vi "Autonomous Independent.vi"() -> ()   [LabVIEW 2012]
doc: "This VI is called when autonomous begins, and will automatically be terminated when autonomous ends. You can carry out timed or sensor driven robot movement independently without needing to return to the caller."
uses:
  AutoInstruction.ctl
  AutoInstructArray.ctl
  Sally_Dashboard_2013/DBNameEnum.ctl
  Robot Global Data.vi
  AutoEnum.ctl
panel:
  in  "DefaultBackupAuto":dbl[](array[numeric])=[2390.0, 30.0, 3.0, 4.0, 1000.0, 0.0]
  in  "AutoBackup":T1
  in  "AutoDefault":T1=[{"Distance/Angle"=30.0, "Speed"=2390.0, "Action"=enum."Aim", "NumFrisbees"=0}, {"Distance/Angle"=5.0, "Speed"=0.0, "Action"=enum."Wait", "NumFrisbees"=0}, {"Distance/Angle"=0.0, "Speed"=0.0, "Action"=enum."Shoot", "NumFrisbees"=4}]
  out "ValueFromDashboard":T1
  in  "Desired steady state (no PID)":dbl=0.5
  in  "Use PID AutoDrive":bool=TRUE
  in  "AutoInstructArray":T1=[{"Distance/Angle"=0.0, "Speed"=0.0, "Action"=enum."DriveForward", "NumFrisbees"=0}, {"Distance/Angle"=0.0, "Speed"=0.0, "Action"=enum."DriveForward", "NumFrisbees"=0}, {"Distance/Angle"=0.0, "Speed"=0.0, "Action"=enum."DriveForward", "NumFrisbees"=0}]
  in  "Instructions":T3(array[cluster])
  in  "Instruction Sequence":T4(array[cluster])
  in  "AutoInstruction":T2
  # "GLENN'S STUFF"
  # "ENUMS FOR\nSTRING UNFLATTENING"
  # "RPM"
  # "Angle"
  # "Wait (s)"
  # "ShootNum"
  # "Time (ms)"
  # "Drive Back Stuff"
  # "Motor Value"
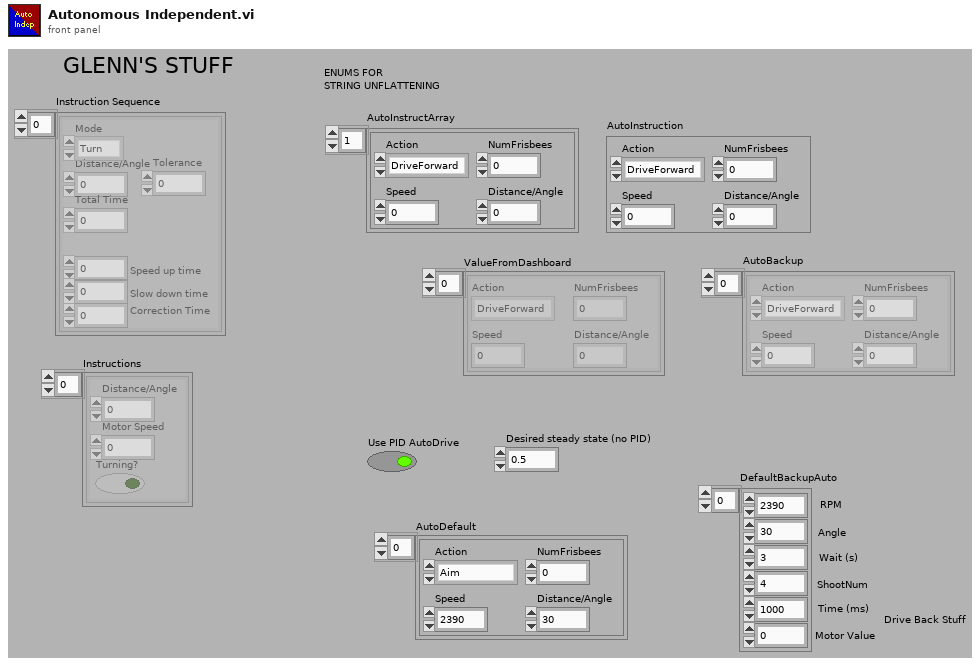
[diagram p1: front panel]
types:
  T1 = typedef "AutoInstructArray.ctl" = T2[]
  T2 = typedef "AutoInstruction.ctl" = cluster{"Distance/Angle":dbl, "Speed":dbl, "Action":enum16{"DriveForward", "Turn", "Aim", "Shoot", "Wait"}, "NumFrisbees":i32}
  T3 = cluster{"Distance/Angle":dbl, "Motor Speed":dbl, "Turning?":bool}[]
  T4 = cluster{"Distance/Angle":dbl, "Tolerance":dbl, "Total Time":dbl, "Mode":enum16{"Turn", "Drive"}, "Correction Time":dbl, "Speed up time":dbl, "Slow down time":dbl}[]
  T5 = typedef "DBNameEnum.ctl" = enum16{"AutoInstructions", "DriveLoopTime", "DriveAlignLSLeft", "DriveAlignLSRight", "Use2DriveAlign", "ClimbLS", "LauncherAngleMatches", "FrameworkVersion", "sLauncherAngle", "LauncherTargetAngle", "sLauncherRPM", "LauncherTargetRPM", "sDriveDistance", "LauncherMotorValue", "PullbackTol", "FireTol", "LauncherRPMTol", "LauncherAngleTol", "InitialWait", "WaitBetweenLaunch", "AnglePresets", "RPMPresets", "UseAngleEncoder", "UseLauncherEncoder", "UseLauncherPID", "QSWaitBeforeFire", "QSWaitBeforeRetract", "AngleForwardValue", "AngleBackwardValue", "UseClusterArray", "BackupAuto", "ReverseDriveIndicate", "HalfSpeedFactor"}
  T6 = typedef "WPI_EncoderDevRef.ctl" = cluster{"DevStatus":errorcluster, "EncoderIndex":T7, "CounterIndex":T8, "DistancePerCount":dbl, "Decoding Type":T9}
  T7 = typedef "FPGA_EncoderIdx.ctl" = enum8{"Enc 0", "Enc 1", "Enc 2", "Enc 3", "Invalid"}
  T8 = typedef "FPGA_CounterCtrSystemIndex.ctl" = enum8{"Ctr 0", "Ctr 1", "Ctr 2", "Ctr 3", "Ctr 4", "Ctr 5", "Ctr 6", "Ctr 7", "Invalid"}
  T9 = typedef "WPI_EncoderType.ctl" = enum16{"1x", "2x", "4x"}
  T10 = typedef "WPI_GyroDevRef.ctl" = cluster{"DevStatus":errorcluster, "Analog Module":T11, "Analog Channel":T12, "Offset":dbl, "Gain (VoltsPerDegree/Second)":dbl}
  T11 = typedef "FPGA_TypedefAnalogModule.ctl" = enum16{"Analog Module 1", "Analog Module 2"}
  T12 = typedef "FPGA_AIChannel.ctl" = enum8{"AI 1", "AI 2", "AI 3", "AI 4", "AI 5", "AI 6", "AI 7", "AI 8", "Invalid"}
  T13 = typedef "WPI_RobotDriveDevRef.ctl" = cluster{"DevStatus":errorcluster, "Motors[]":T14[], "Square Inputs":bool, "Max Output":dbl, "Isochronous":bool}
  T14 = typedef "WPI_MotorControlDeviceRef.ctl" = cluster{"DeviceStatus":errorcluster, "Type":enum16{"PWM", "CAN"}, "PWM":cluster{"Digital Module":T15, "PWM Channel":T16, "DeadBand":T17}, "CAN":cluster{"Device Number":u8, "Control Mode":T18, "Semaphore":T19, "Max Vout":dbl}, "Invert":bool, "TransformRef":T20, "InvTransformRef":T20}
  T15 = typedef "FPGA_TypedefDigitalModule.ctl" = enum16{"Digital Module 1", "Digital Module 2"}
  T16 = typedef "FPGA_DIOPWMChannel.ctl" = enum8{"PWM 1", "PWM 2", "PWM 3", "PWM 4", "PWM 5", "PWM 6", "PWM 7", "PWM 8", "PWM 9", "PWM 10", "Invalid"}
  T17 = typedef "WPI_PWMDeadband.ctl" = cluster{"Name":string, "maxPositivePwm":i32, "minPositivePwm":i32, "centerPwm":i32, "maxNegativePwm":i32, "minNegativePwm":i32, "angularRange":u16}
  T18 = typedef "WPI_CANJaguar_ControlMode.ctl" = enum8{"Percent VBus", "Current", "Speed", "Position", "Voltage"}
  T19 = typedef "Semaphore RefNum" = refnum<k1>
  T20 = typedef "WPI_PWMTransform_ConPane.ctl" = refnum<vi>
  T21 = typedef "AutoEnum.ctl" = enum16{"Disabled", "BackRight", "BackLeft", "CloseRight", "CloseLeft", "BehindPyramid"}
  T22 = enum16{"DriveForward", "Turn", "Aim", "Shoot", "Wait", "LauncherDown"}
  T23 = enum16{"DriveForward", "Turn", "Aim", "Shoot", "Wait"}
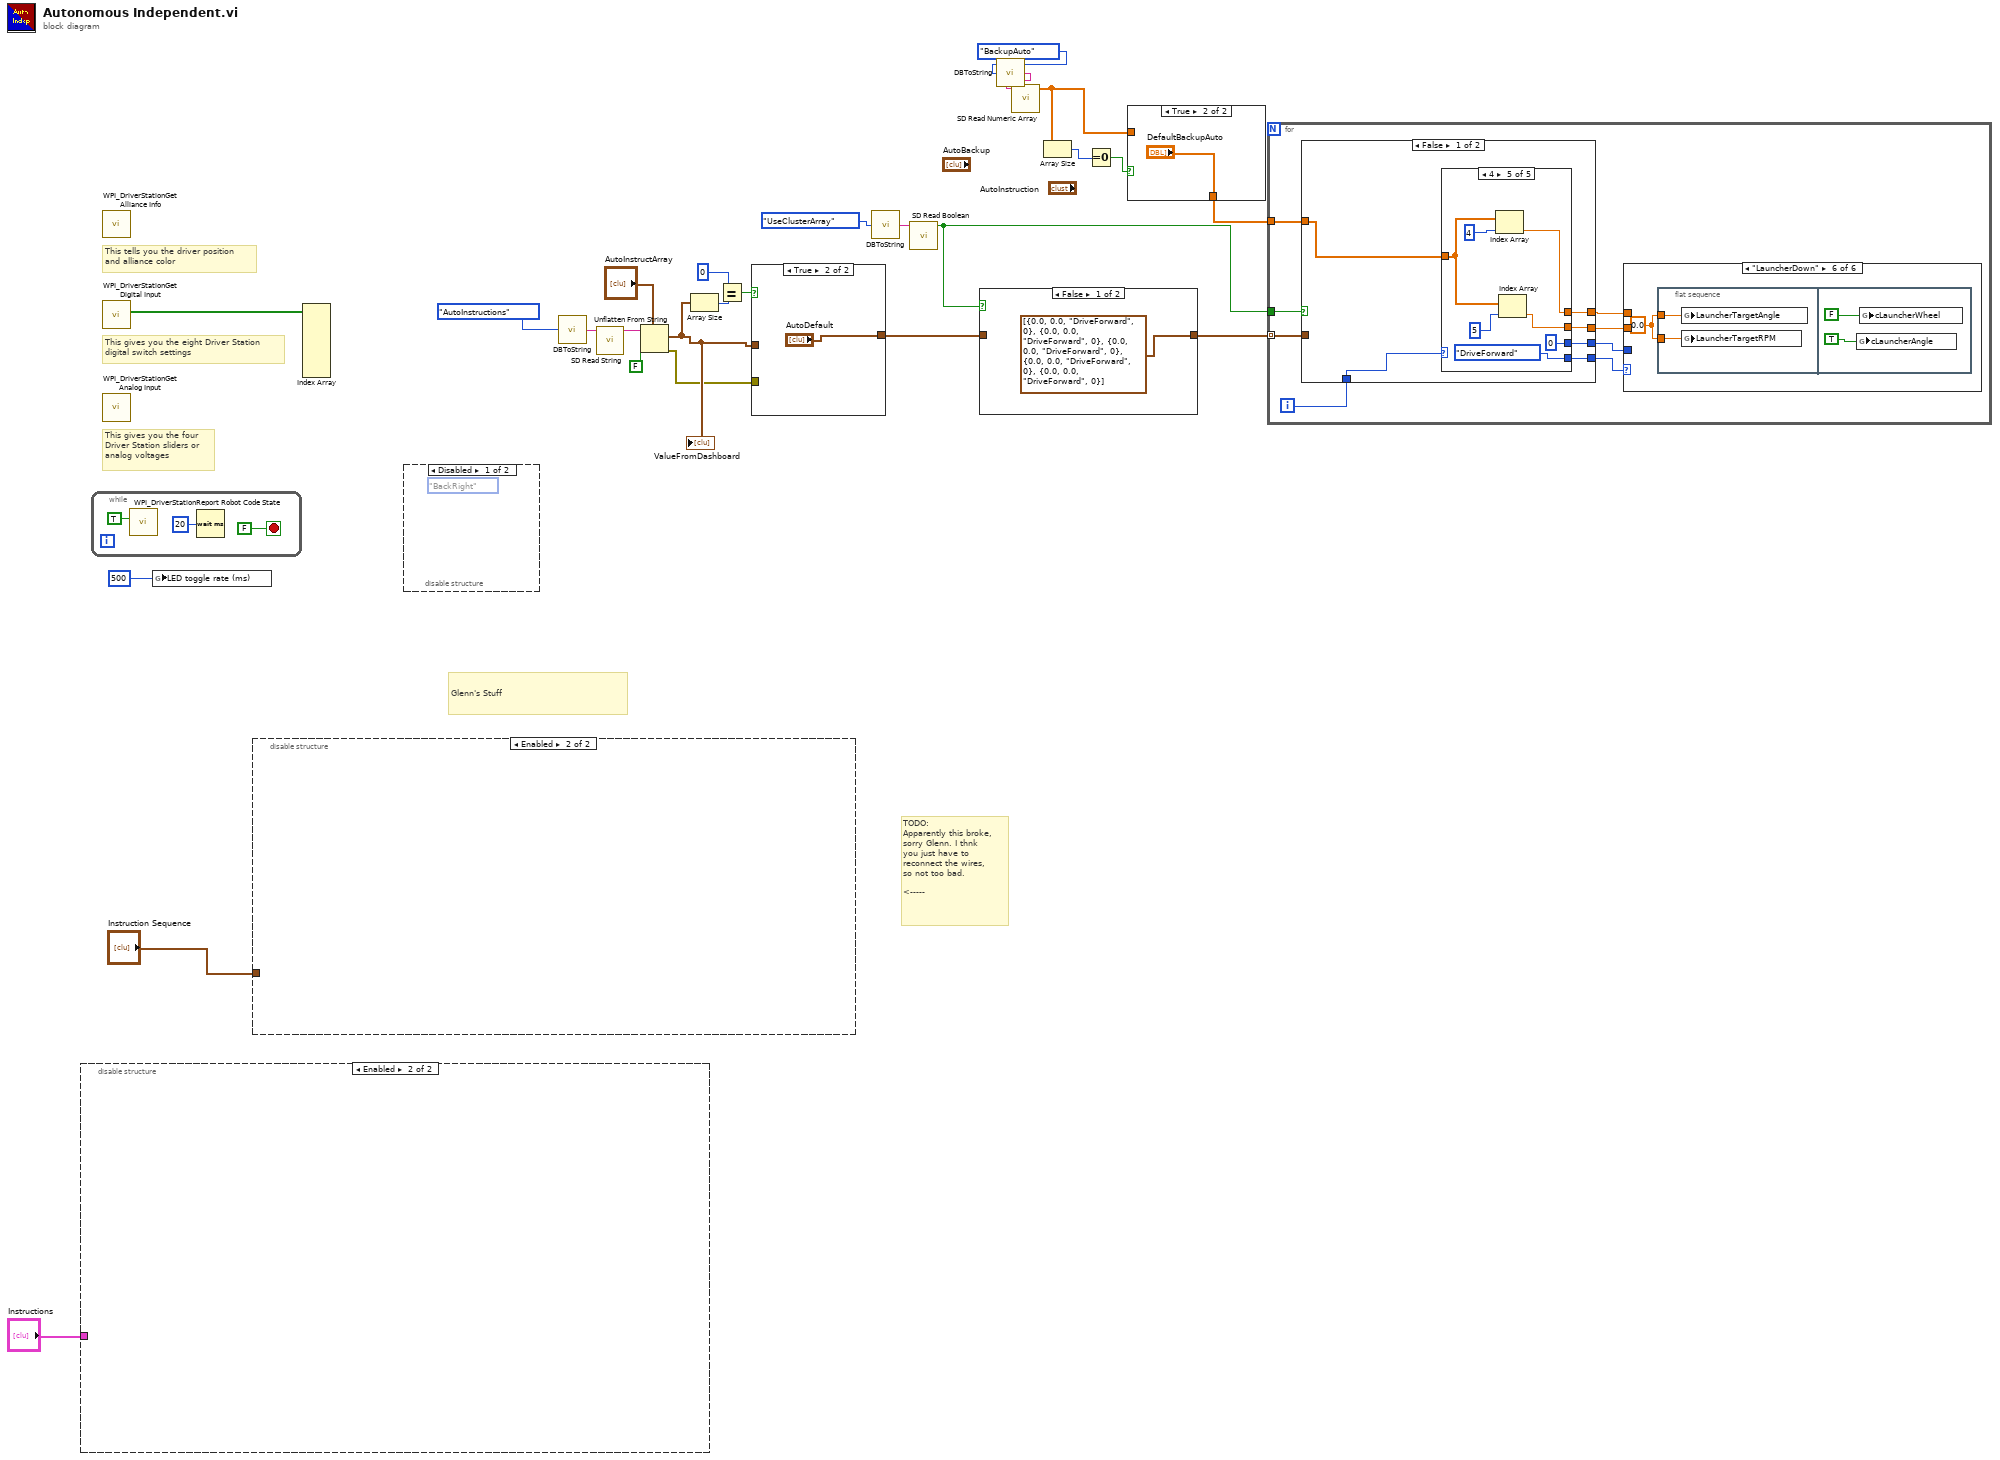
[diagram p0: block diagram]
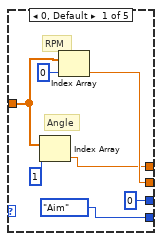
[diagram p5: hidden frame]
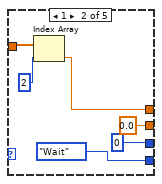
[diagram p6: hidden frame]
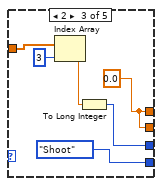
[diagram p7: hidden frame]
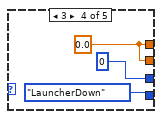
[diagram p8: hidden frame]
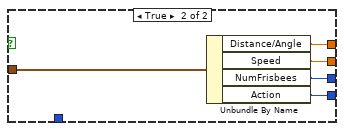
[diagram p9: hidden frame]
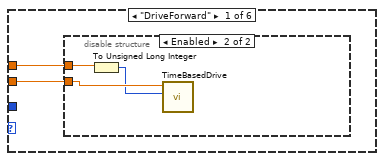
[diagram p10: hidden frame]
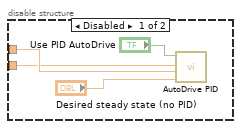
[diagram p11: hidden frame]
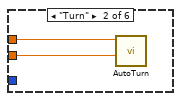
[diagram p12: hidden frame]
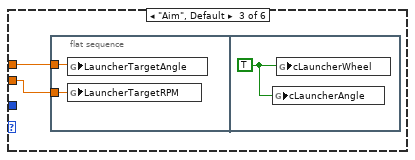
[diagram p13: hidden frame]
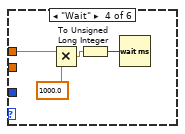
[diagram p14: hidden frame]
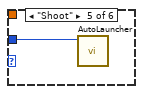
[diagram p15: hidden frame]
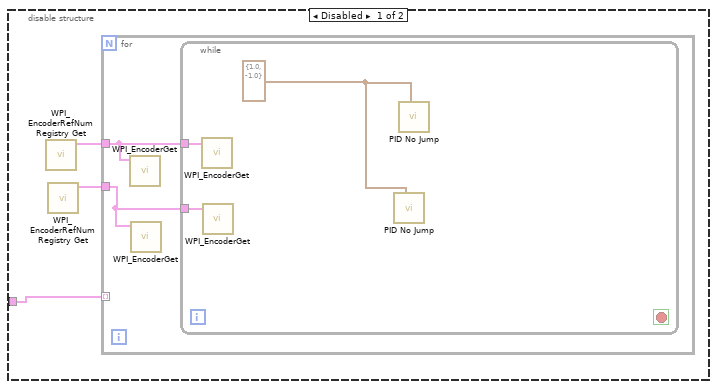
[diagram p17: hidden frame]
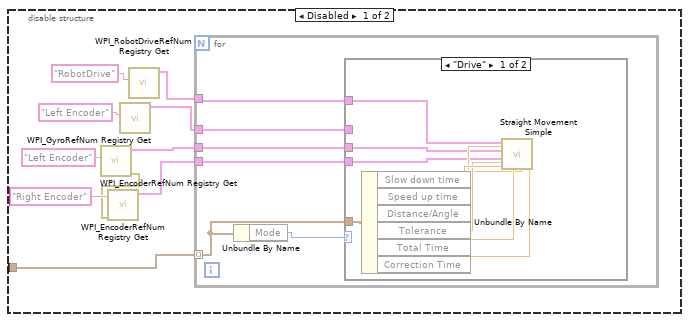
[diagram p18: hidden frame]
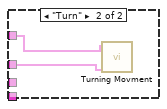
[diagram p19: hidden frame]
diagram:
  # "TODO:\nApparently this broke,\nsorry Glenn. I thnk\nyou just have to\nreconnect the wires,\nso not too bad.\n\n<-----"
  # "Glenn's Stuff"
  # "This tells you the driver position\nand alliance color"
  # "This gives you the eight Driver Station\ndigital switch settings"
  # "This gives you the four\nDriver Station sliders or\nanalog voltages"
  n1 = disable-structure shown="Enabled" {
    disable-tunnel: "Instructions" -> [w26 _]
    frame Disabled {
      n2 = call <vilib>:"WPI_EncoderRefNum Registry Get.vi"() -> ("EncoderDevRef"=w28:T6)  [unwired: 10 in, 1 out]
      n3 = call <vilib>:"WPI_EncoderRefNum Registry Get.vi"() -> ("EncoderDevRef"=w27:T6)  [unwired: 10 in, 1 out]
      n4 = for {
        tunnel: w28 -> [w30]
        tunnel: w27 -> [w29]
        tunnel: w26 -> [_] mode=indexing
        n5 = call <vilib>:"WPI_EncoderGet.vi"("EncoderDevRef"=w30) -> ()  [unwired: 5 in, 6 out]
        n6 = call <vilib>:"WPI_EncoderGet.vi"("EncoderDevRef"=w29) -> ()  [unwired: 5 in, 6 out]
        n7 = while {
          tunnel: w30 -> [w32]
          tunnel: w29 -> [w33]
          stop <- _ stop-if-true
          w31 = cluster{"output high":dbl, "output low":dbl} {"output high"=1.0, "output low"=-1.0} ("output range")
          n8 = call <vilib>:"WPI_EncoderGet.vi"("EncoderDevRef"=w32) -> ()  [unwired: 5 in, 6 out]
          n9 = call <vilib>:"WPI_EncoderGet.vi"("EncoderDevRef"=w33) -> ()  [unwired: 5 in, 6 out]
          n10 = call "PID No Jump.vi"("output range"=w31) -> ()  [unwired: 10 in, 1 out]
          n11 = call "PID No Jump.vi"("output range"=w31) -> ()  [unwired: 10 in, 1 out]
        }
      }
    }
    frame Enabled {
    }
  }
  n12 = while {
    stop <- FALSE stop-if-true
    n13 = call <vilib>:"WPI_DriverStationReport Robot Code State.vi"("Autonomous"=TRUE) -> ()  [unwired: 10 in, 1 out]
    n14 = Wait (ms)(milliseconds to wait=u32 20) -> ()  [unwired: 1 out]
  }
  n15 = call <vilib>:"WPI_DriverStationGet Alliance Info.vi"() -> ()  [unwired: 12 out]
  n16 = call <vilib>:"WPI_DriverStationGet Digital Input.vi"() -> ("Driver Station Digital Input (1-8)"=w25:bool[])  [unwired: 11 out]
  n17 = call <vilib>:"WPI_DriverStationGet Analog Input.vi"() -> ()  [unwired: 12 out]
  n18 = global write "Robot Global Data.vi" "LED toggle rate (ms)"(u32 500 ("LED ms toggle rate")) -> ()
  n19 = disable-structure shown="Enabled" {
    disable-tunnel: "Instruction Sequence" -> [w46 _]
    frame Disabled {
      n20 = call <vilib>:"WPI_EncoderRefNum Registry Get.vi"("refnum name"="Left Encoder") -> ("error out"=w37:errorcluster, "EncoderDevRef"=w43:T6)  [unwired: 9 in]
      n21 = call <vilib>:"WPI_EncoderRefNum Registry Get.vi"("error in (no error)"=w37, "refnum name"="Right Encoder") -> ("EncoderDevRef"=w42:T6)  [unwired: 8 in, 1 out]
      n22 = call <vilib>:"WPI_GyroRefNum Registry Get.vi"("refnum name"="Left Encoder") -> ("GyroDevRef"=w44:T10)  [unwired: 9 in, 1 out]
      n23 = call <vilib>:"WPI_RobotDriveRefNum Registry Get.vi"("refnum name"="RobotDrive") -> ("RobotDriveDevRef"=w45:T13)  [unwired: 9 in, 1 out]
      n24 = for {
        tunnel: w46 -> [w51] mode=indexing
        tunnel: w45 -> [w50]
        tunnel: w44 -> [w49]
        tunnel: w43 -> [w48]
        tunnel: w42 -> [w47]
        n25 = Unbundle By Name(w51) -> ("Mode"=w52:enum16{"Turn", "Drive"})
        n26 = case shown="\"Drive\"" w52 {
          tunnel: w51 -> [w62 _]
          tunnel: w50 -> [w55 w64]
          tunnel: w49 -> [_ w63]
          tunnel: w48 -> [w54 _]
          tunnel: w47 -> [w53 _]
          frame "Drive" {
            n27 = Unbundle By Name(w62) -> ("Slow down time"=w57:dbl, "Speed up time"=w56:dbl, "Distance/Angle"=w61:dbl, "Tolerance"=w60:dbl, "Total Time"=w59:dbl, "Correction Time"=w58:dbl)
            n28 = call "Straight Movement Simple.vi"(0:w58, 4:w60, 5:w57, 6:w59, 7:w56, 8:w61, 9:w53, 10:w54, 11:w55) -> ()  [unwired: 2 in, 1 out]
          }
          frame "Turn" {
            n29 = call "Turning Movment.vi"("GyroDevRef"=w63, "RobotDriveDevRef"=w64) -> ()  [unwired: 9 in, 1 out]
          }
        }
      }
    }
    frame Enabled {
    }
  }
  n30 = Index Array(array=w25) -> ()  [unwired: 8 in, 8 out]
  n31 = disable-structure shown="Disabled" {
    frame Disabled {
      (unwired) AutoEnum."BackRight" ("AutoEnum")
    }
    frame Enabled {
    }
  }
  n32 = call "DBToString.vi"("Enum"=DBNameEnum."AutoInstructions") -> ("Refname"=w15:string)
  n33 = call <vilib>:"SD Read String.vi"("Name"=w15) -> ("String"=w14:string)  [unwired: 8 in, 2 out]
  n34 = Unflatten From String(type="AutoInstructArray", binary string=w14, data includes array or string size? (T)=FALSE) -> (value=w17:T1, error out=w13:errorcluster)  [unwired: 2 in, 1 out]
  "ValueFromDashboard" <- w17
  n35 = Array Size(array=w17) -> (size(s)=w20:i32)
  n36 = Equal?(x=w20, y=0) -> (x = y?=w18:bool)
  n37 = case shown="True" w18 {
    tunnel: w17 -> [w65 _]
    tunnel: [w65 "AutoDefault"] -> w9
    tunnel: w13 -> [_ _]
    frame False {
    }
    frame True {
    }
  }
  n38 = call "DBToString.vi"("Enum"=DBNameEnum."UseClusterArray") -> ("Refname"=w11:string)
  n39 = call <vilib>:"SD Read Boolean.vi"("Name"=w11) -> ("Boolean"=w8:bool)  [unwired: 8 in, 2 out]
  n40 = case shown="False" w8 {
    tunnel: w9 -> [_ w68]
    tunnel: [T1 [{"Distance/Angle"=0.0, "Speed"=0.0, "Action"=enum."DriveForward", "NumFrisbees"=0}, {"Distance/Angle"=0.0, "Speed"=0.0, "Action"=enum."DriveForward", "NumFrisbees"=0}, {"Distance/Angle"=0.0, "Speed"=0.0, "Action"=enum."DriveForward", "NumFrisbees"=0}, {"Distance/Angle"=0.0, "Speed"=0.0, "Action"=enum."DriveForward", "NumFrisbees"=0}, {"Distance/Angle"=0.0, "Speed"=0.0, "Action"=enum."DriveForward", "NumFrisbees"=0}] ("AutoBackup 2") w68] -> w7
    frame False {
    }
    frame True {
    }
  }
  n41 = call "DBToString.vi"("Enum"=DBNameEnum."BackupAuto") -> ("Refname"=w6:string)
  n42 = call <vilib>:"SD Read Numeric Array.vi"("Name"=w6) -> ("Numeric Array"=w1:dbl[])  [unwired: 8 in, 2 out]
  n43 = Array Size(array=w1) -> (size(s)=w3:i32)
  n44 = Equal To 0?(x=w3) -> (x = 0?=w2:bool)
  n45 = case shown="True" w2 {
    tunnel: w1 -> [w69 _]
    tunnel: [w69 "DefaultBackupAuto"] -> w4
    frame False {
    }
    frame True {
    }
  }
  n46 = for {
    tunnel: w7 -> [w74] mode=indexing
    tunnel: w8 -> [w73]
    tunnel: w4 -> [w71]
    i -> [w72]
    n47 = case shown="False" w73 {
      tunnel: [w81 w118] -> w78
      tunnel: [w82 w117] -> w77
      tunnel: [w83 w116] -> w76
      tunnel: [w80 w115] -> w75
      tunnel: w74 -> [_ w114]
      tunnel: w72 -> [w84 _]
      tunnel: w71 -> [w79 _]
      frame False {
        n48 = case shown="4" w84 {
          tunnel: w79 -> [w90 w97 w103 _ w111]
          tunnel: [T22."Aim" ("Action") T22."Wait" ("Action") T22."Shoot" ("Action") T22."LauncherDown" ("Action") T22."DriveForward" ("Action")] -> w83
          tunnel: [w88 0.0 ("Numeric") w99 w106 w109] -> w82
          tunnel: [w87 w95 w99 w106 w110] -> w81
          tunnel: [0 0 w100 0 0] -> w80
          frame 0, Default {
            # "RPM"
            # "Angle"
            n49 = Index Array(array=w90, index=1) -> (element=w87:dbl)
            n50 = Index Array(array=w90, index=0) -> (element=w88:dbl)
          }
          frame 1 {
            n51 = Index Array(array=w97, index=2) -> (element=w95:dbl)
          }
          frame 2 {
            w99 = 0.0 ("Numeric")
            n52 = Index Array(array=w103, index=3) -> (element=w101:dbl)
            n53 = To Long Integer(number=w101) -> (32bit integer=w100:i32)
          }
          frame 3 {
            w106 = 0.0 ("Numeric")
          }
          frame 4 {
            n54 = Index Array(array=w111, index=4) -> (element=w110:dbl)
            n55 = Index Array(array=w111, index=5) -> (element=w109:dbl)
          }
        }
      }
      frame True {
        n56 = Unbundle By Name(w114) -> ("Distance/Angle"=w118:dbl, "Speed"=w117:dbl, "NumFrisbees"=w115:i32, "Action"=w116:T23)
      }
    }
    n57 = case shown="\"LauncherDown\"" w76 {
      tunnel: w78 -> [w120 w129 w131 w137 _ _]
      tunnel: w77 -> [w119 w128 w130 _ _ _]
      tunnel: w75 -> [_ _ _ _ w139 _]
      frame "DriveForward" {
        n58 = disable-structure shown="Enabled" {
          disable-tunnel: w120 -> [w124 w126]
          disable-tunnel: w119 -> [w121 w127]
          frame Disabled {
            n59 = call "AutoDrive PID.vi"("Steady Val (no PID only)"="Desired steady state (no PID)", "Distance to travel (inches)"=w124, "Desired RPM (PID only)"=w121, "Use PID"="Use PID AutoDrive") -> ()  [unwired: 8 in]
          }
          frame Enabled {
            n60 = To Unsigned Long Integer(number=w126) -> (unsigned 32bit integer=w125:u32)
            n61 = call "TimeBasedDrive.vi"("Time (ms)"=w125, "Motor Value"=w127) -> ()  [unwired: 10 in]
          }
        }
      }
      frame "Turn" {
        n62 = call "AutoTurn.vi"("Steady Val"=w128, "Degrees to turn"=w129) -> ()  [unwired: 10 in]
      }
      frame "Aim", Default {
        n63 = flat-sequence {
          tunnel: w131 -> [w133]
          tunnel: w130 -> [w132]
          frame #0 {
            n64 = global write "Robot Global Data.vi" "LauncherTargetAngle"(w133) -> ()
            n65 = global write "Robot Global Data.vi" "LauncherTargetRPM"(w132) -> ()
          }
          frame #1 {
            w134 = TRUE ("cLauncherWheel")
            n66 = global write "Robot Global Data.vi" "cLauncherAngle"(w134) -> ()
            n67 = global write "Robot Global Data.vi" "cLauncherWheel"(w134) -> ()
          }
        }
      }
      frame "Wait" {
        n68 = Multiply(x=w137, y=1000.0) -> (x*y=w136:dbl)
        n69 = To Unsigned Long Integer(number=w136) -> (unsigned 32bit integer=w135:u32)
        n70 = Wait (ms)(milliseconds to wait=w135) -> ()  [unwired: 1 out]
      }
      frame "Shoot" {
        n71 = call "AutoLauncher.vi"("# Frisbees"=w139) -> ()  [unwired: 11 in]
      }
      frame "LauncherDown" {
        w140 = 0.0
        n72 = flat-sequence {
          tunnel: w140 -> [w142]
          tunnel: w140 -> [w141]
          frame #0 {
            n73 = global write "Robot Global Data.vi" "LauncherTargetAngle"(w142) -> ()
            n74 = global write "Robot Global Data.vi" "LauncherTargetRPM"(w141) -> ()
          }
          frame #1 {
            n75 = global write "Robot Global Data.vi" "cLauncherAngle"(TRUE ("cLauncherWheel")) -> ()
            n76 = global write "Robot Global Data.vi" "cLauncherWheel"(FALSE ("cLauncherWheel")) -> ()
          }
        }
      }
    }
  }
